vi "Do Operation - Use Dynamic Dispatch Method.vi"(8 "error in (no error)":errorcluster, 11 "Cluster With Class":T1) -> (0 "error out":errorcluster, 3 "Cluster With Class Out":T1)   [LabVIEW 2012]
uses:
  ClassDefinitions/SimpleClassWithMethods/SimpleArithmetic.lvclass
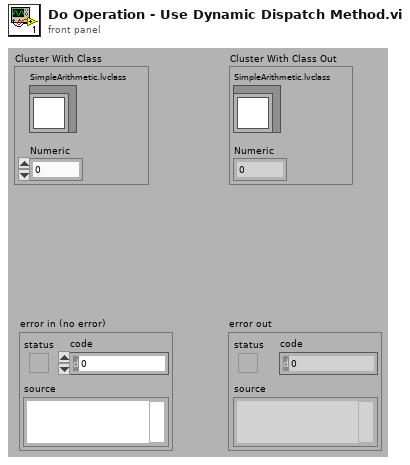
[diagram p1: front panel]
types:
  T1 = cluster{"SimpleArithmetic.lvclass":refnum<class "SimpleArithmetic.lvclass">, "Numeric":dbl}
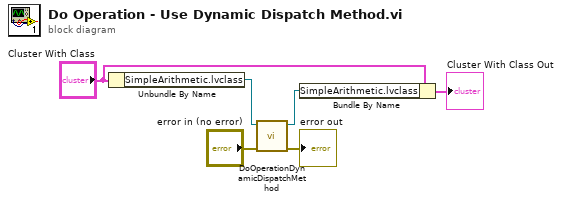
[diagram p0: block diagram]
diagram:
  n1 = Unbundle By Name("Cluster With Class") -> ("SimpleArithmetic.lvclass"=w4:refnum<class "SimpleArithmetic.lvclass">)
  n2 = call-dynamic "DoOperationDynamicDispatchMethod.vi"("error in (no error)"="error in (no error)", "SimpleArithmetic in"=w4) -> ("error out"=→"error out":errorcluster, "SimpleArithmetic out"=w3:refnum<class "SimpleArithmetic.lvclass">)  [unwired: 8 in]
  n3 = Bundle By Name(cluster="Cluster With Class", "SimpleArithmetic.lvclass"=w3) -> (→"Cluster With Class Out":T1)
